vi "SGSA_Sweep_ALL_Ch.vi"() -> ()   [LabVIEW 2023, in "SG_SA.lvlib"]
uses:
  SG_SA.lvlib
  Clover_Cell.lvlib
panel:
  out "Channel No.":i32
  in  "Polarity":u16(ring)=1 items=["V", "H"]
  in  "TRXmod":u16(ring)=1 items=["Rx"=2, "Tx"=1]
  in  "FileNote":string
  out "SG Power":i32
  in  "Stop Power":i32=8
  in  "Start Power":i32=-40
  in  "SG":refnum<visa-resource-name>="TCPIP::192.168.100.200::inst0::INSTR"
  in  "AvgTimes":i32=10
  in  "SA":refnum<visa-resource-name>="TCPIP::192.168.100.230::inst0::INSTR"
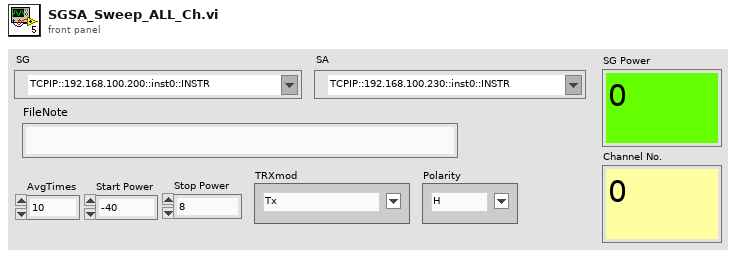
[diagram p1: front panel]
types:
  T1 = cluster{"Mode":u16, "Polarity":u16, "CH_ON/OFF":u16, "Channel":i32, "Gain":i32, "Phase":i32}
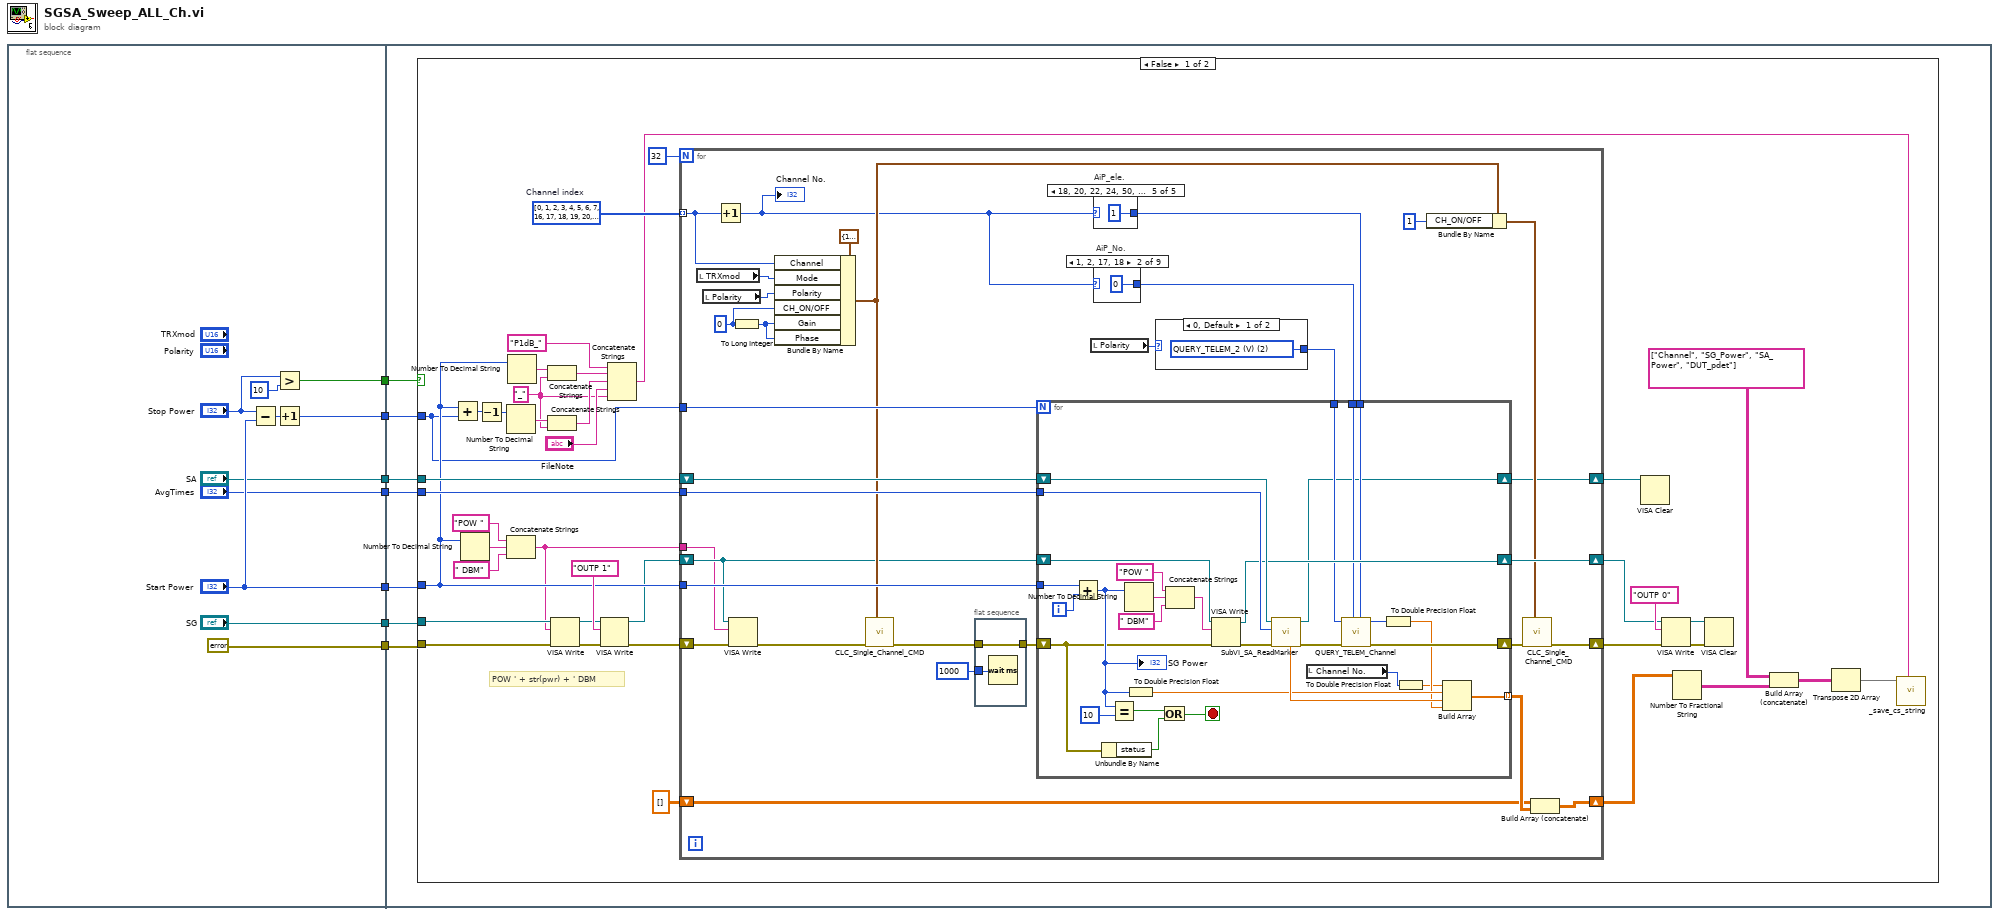
[diagram p0: block diagram]
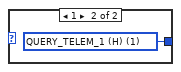
[diagram p2: hidden frame]
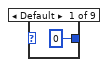
[diagram p3: hidden frame]
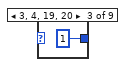
[diagram p4: hidden frame]
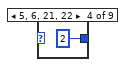
[diagram p5: hidden frame]
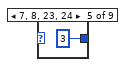
[diagram p6: hidden frame]
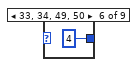
[diagram p7: hidden frame]
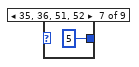
[diagram p8: hidden frame]
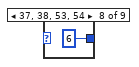
[diagram p9: hidden frame]
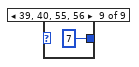
[diagram p10: hidden frame]
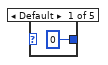
[diagram p11: hidden frame]
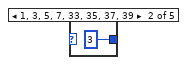
[diagram p12: hidden frame]
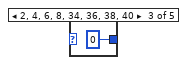
[diagram p13: hidden frame]
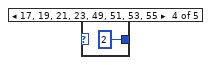
[diagram p14: hidden frame]
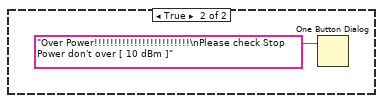
[diagram p15: hidden frame]
diagram:
  n1 = flat-sequence {
    tunnel: ["SA"] -> w7
    tunnel: [errorcluster {"status"=FALSE, "code"=0, "source"=""} ("error in (no error)")] -> w6
    tunnel: ["SG"] -> w5
    tunnel: [w12] -> w4
    tunnel: ["Start Power"] -> w3
    tunnel: ["AvgTimes"] -> w2
    tunnel: [w13] -> w1
    tunnel: w7 -> [w24]
    tunnel: w6 -> [w23]
    tunnel: w5 -> [w22]
    tunnel: w4 -> [w21]
    tunnel: w3 -> [w20]
    tunnel: w2 -> [w19]
    tunnel: w1 -> [w18]
    frame #0 {
      n2 = Subtract(x="Stop Power", y="Start Power") -> (x-y=w16:i32)
      n3 = Greater?(x="Stop Power", y=10) -> (0:w12:bool)
      n4 = Increment(x=w16) -> (x+1=w13:i32)
    }
    frame #1 {
      n5 = case shown="False" w21 {
        tunnel: w24 -> [w63 _]
        tunnel: w19 -> [w62 _]
        tunnel: w20 -> [w43 _]
        tunnel: w23 -> [w46 _]
        tunnel: w22 -> [w45 _]
        tunnel: w18 -> [w42 _]
        frame False {
          w36 = i32[] [0, 1, 2, 3, 4, 5, 6, 7, 16, 17, 18, 19, 20, 21, 22, 23, 32, 33, 34, 35, 36, 37, 38, 39, 48, 49, 50, 51, 52, 53, 54, 55]  # Channel index
          w38 = "_"
          # "POW ' + str(pwr) + ' DBM"
          n6 = Add(x=w43, y=w42) -> (x+y=w57:i32)
          n7 = Number To Decimal String(number=w43) -> (decimal integer string=w48:string)  [unwired: 1 in]
          n8 = Decrement(x=w57) -> (x-1=w56:i32)
          n9 = Number To Decimal String(number=w56) -> (decimal integer string=w54:string)  [unwired: 1 in]
          n10 = Concatenate Strings("POW ", w48, " DBM") -> (w35:string)
          n11 = Number To Decimal String(number=w43) -> (decimal integer string=w55:string)  [unwired: 1 in]
          n12 = Concatenate Strings(w55, w38) -> (w52:string)
          n13 = Concatenate Strings(w54, w38) -> (w51:string)
          n14 = VISA Write(VISA resource name=w45, write buffer=w35, error in (no error)=w46) -> (VISA resource name out=w44:refnum<visa-resource-name>, error out=w47:errorcluster)  [unwired: 1 out]
          n15 = VISA Write(VISA resource name=w44, write buffer="OUTP 1", error in (no error)=w47) -> (VISA resource name out=w41:refnum<visa-resource-name>, error out=w61:errorcluster)  [unwired: 1 out]
          n16 = Concatenate Strings("P1dB_" ("delimiter (\\t)"), w52, w51, "FileNote", w38) -> (w33:string)
          n17 = for {
            N: 32 -> [_]
            tunnel: w62 -> [w94]
            tunnel: w43 -> [w93]
            tunnel: w42 -> [w92]
            shift-right: [w79] -> w58
            shift-left: w61 -> [w74]
            shift-right: [w91] -> w40
            shift-left: w41 -> [w73]
            tunnel: w36 -> [w85] mode=indexing
            tunnel: w35 -> [w72]
            shift-right: [w69] -> w30
            shift-left: dbl[][] [] -> [w68]
            shift-right: [w67] -> w25
            shift-left: w63 -> [w95]
            w87 = u16 0 ("CH_ON/OFF")
            n18 = local read "TRXmod"() -> (w88:u16)
            n19 = local read "Polarity"() -> (w89:u16)
            n20 = Increment(x=w85) -> (x+1=w75:i32)
            "Channel No." <- w75
            n21 = VISA Write(VISA resource name=w73, write buffer=w72, error in (no error)=w74) -> (error out=w65:errorcluster)  [unwired: 2 out]
            n22 = To Long Integer(number=w87) -> (32bit integer=w90:i32)
            n23 = Bundle By Name(cluster=T1 {"Mode"=1, "Polarity"=1, "CH_ON/OFF"=1, "Channel"=0, "Gain"=0, "Phase"=0} ("Channel params"), "Channel"=w85, "Mode"=w88, "Polarity"=w89, "CH_ON/OFF"=w87, "Gain"=w90, "Phase"=w90) -> (w77:T1)
            n24 = call "CLC_Single_Channel_CMD.vi"("Channel params"=w77, "error in"=w65) -> ("error out"=w64:errorcluster)  [unwired: 7 in, 2 out]
            n25 = flat-sequence {
              tunnel: w64 -> [w97]
              tunnel: [w97] -> w66
              tunnel: u32 1000 ("milliseconds to wait") -> [w96]
              frame #0 {
                n26 = Wait (ms)(milliseconds to wait=w96) -> ()  [unwired: 1 out]
              }
            }
            n27 = local read "Polarity"() -> (w84:u16)
            n28 = case "AiP_ele." shown="18, 20, 22, 24, 50, 52, 54, 56" w75 {
              tunnel: [0 3 0 2 1] -> w83
              frame Default {
              }
              frame 1, 3, 5, 7, 33, 35, 37, 39 {
              }
              frame 2, 4, 6, 8, 34, 36, 38, 40 {
              }
              frame 17, 19, 21, 23, 49, 51, 53, 55 {
              }
              frame 18, 20, 22, 24, 50, 52, 54, 56 {
              }
            }
            n29 = case "AiP_No." shown="1, 2, 17, 18" w75 {
              tunnel: [0 0 1 2 3 4 5 6 7] -> w82
              frame Default {
              }
              frame 1, 2, 17, 18 {
              }
              frame 3, 4, 19, 20 {
              }
              frame 5, 6, 21, 22 {
              }
              frame 7, 8, 23, 24 {
              }
              frame 33, 34, 49, 50 {
              }
              frame 35, 36, 51, 52 {
              }
              frame 37, 38, 53, 54 {
              }
              frame 39, 40, 55, 56 {
              }
            }
            n30 = case shown="0, Default" w84 {
              tunnel: [w98 w99] -> w81
              frame 0, Default {
                w98 = u16 2 items=["QUERY_TELEM_2 (V)"=2, "QUERY_TELEM_1 (H)"=1] ("TRXmode")
              }
              frame 1 {
                w99 = u16 1 items=["QUERY_TELEM_2 (V)"=2, "QUERY_TELEM_1 (H)"=1] ("TRXmode")
              }
            }
            n31 = for {
              N: w92 -> [_]
              tunnel: w94 -> [w142]
              tunnel: w93 -> [w139]
              shift-right: [w128] -> w80
              shift-left: w66 -> [w117]
              shift-right: [w125] -> w91
              shift-left: w73 -> [w124]
              tunnel: w83 -> [w123]
              tunnel: w82 -> [w122]
              tunnel: w81 -> [w121]
              tunnel: [w118] -> w70 mode=indexing
              shift-right: [w114] -> w67
              shift-left: w95 -> [w143]
              i -> [w140]
              stop <- w116 stop-if-true
              n32 = Add(x=w139, y=w140) -> (x+y=w132:i32)
              "SG Power" <- w132
              n33 = Unbundle By Name(w117) -> ("status"=w115:bool)
              n34 = Equal?(x=w132, y=10) -> (x = y?=w130:bool)
              n35 = Number To Decimal String(number=w132) -> (decimal integer string=w136:string)  [unwired: 1 in]
              n36 = To Double Precision Float(number=w132) -> (double precision float=w133:dbl)
              n37 = Or(x=w130, y=w115) -> (x .or. y?=w116:bool)
              n38 = Concatenate Strings("POW ", w136, " DBM") -> (w135:string)
              n39 = VISA Write(VISA resource name=w124, write buffer=w135, error in (no error)=w117) -> (VISA resource name out=w125:refnum<visa-resource-name>, error out=w141:errorcluster)  [unwired: 1 out]
              n40 = call "SubVI_SA_ReadMarker.vi"("error in (no error)"=w141, "AvgTimes"=w142, "VISA resource name"=w143) -> ("error out"=w129:errorcluster, "VISA resource name out"=w114:refnum<visa-resource-name>, "Marker Power"=w134:dbl)  [unwired: 5 in, 1 out]
              n41 = local read "Channel No."() -> (w120:i32)
              n42 = call "QUERY_TELEM_Channel.vi"("AiP_ele."=w123, "AiP_No."=w122, "error in"=w129, "TRXmode"=w121) -> ("error out"=w128:errorcluster, "pdet"=w127:i32)  [unwired: 6 in]
              n43 = To Double Precision Float(number=w127) -> (double precision float=w126:dbl)
              n44 = To Double Precision Float(number=w120) -> (double precision float=w119:dbl)
              n45 = Build Array(w119, w133, w134, w126) -> (w118:dbl[])
            }
            n46 = Bundle By Name(cluster=w77, "CH_ON/OFF"=u16 1) -> (w76:T1)
            n47 = call "CLC_Single_Channel_CMD.vi"("Channel params"=w76, "error in"=w80) -> ("error out"=w79:errorcluster)  [unwired: 7 in, 2 out]
            n48 = Build Array (concatenate)(w68, w70) -> (w69:dbl[][])
          }
          n49 = VISA Clear(VISA resource name=w25) -> ()  [unwired: 1 in, 2 out]
          n50 = VISA Write(VISA resource name=w40, write buffer="OUTP 0", error in (no error)=w58) -> (VISA resource name out=w26:refnum<visa-resource-name>, error out=w27:errorcluster)  [unwired: 1 out]
          n51 = Number To Fractional String(number=w30) -> (F-format string=w32:string[][])  [unwired: 3 in]
          n52 = VISA Clear(VISA resource name=w26, error in (no error)=w27) -> ()  [unwired: 2 out]
          n53 = Build Array (concatenate)(string[][] [["Channel", "SG_Power", "SA_Power", "DUT_pdet"]] ("array"), w32) -> (w29:string[][])
          n54 = Transpose 2D Array(2D array=w29) -> (transposed array=w28:string[][])
          n55 = call "_save_cs_string.vi"("FileName"=w33, "Array"=w28) -> ()  [unwired: 9 in, 1 out]
        }
        frame True {
          n56 = One Button Dialog(message="Over Power!!!!!!!!!!!!!!!!!!!!!!!!\nPlease check Stop Power don't over [ 10 dBm ]") -> ()  [unwired: 1 in, 1 out]
        }
      }
    }
  }
